vi "Manual_Motor_Test.vi"(11 "Manual Motor Controll":bool) -> ()   [LabVIEW 2016]
doc: "Drive the motor manually via the H-Bridge using this VI"
panel:
  in  "stopMotors":bool
  in  "direction":enum16{"Forward", "Backward"}(ring)
  in  "motorSelect":enum16{"Motor A", "Motor B"}(ring)
  # "ON"
  # "OFF"
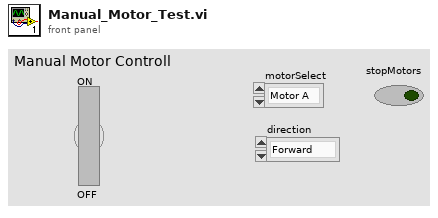
[diagram p1: front panel]
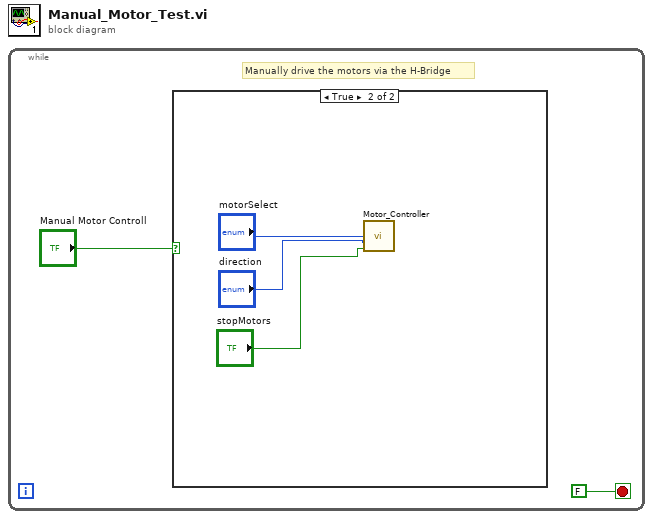
[diagram p0: block diagram]
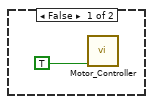
[diagram p2: hidden frame]
diagram:
  n1 = while {
    stop <- FALSE stop-if-true
    # "Manually drive the motors via the H-Bridge"
    n2 = case shown="True" "Manual Motor Controll" {
      frame False {
        n3 = call "Motor_Controller.vi"("stopMotors"=TRUE) -> ()  [unwired: 14 in, 1 out]
      }
      frame True {
        n4 = call "Motor_Controller.vi"("motorSelect"="motorSelect", "direction"="direction", "stopMotors"="stopMotors") -> ()  [unwired: 12 in, 1 out]
      }
    }
  }
